vi "Cost.vi"(1 "Y":T1, 2 "Predictions":T1) -> (0 "Cost":dbl)   [LabVIEW 2016]
uses:
  <vilib>/Analysis/Matrix/Datatypes/RealMatrix.ctl
  <vilib>/Analysis/7linalg.llb/Real Transpose Matrix.vi
  <vilib>/Analysis/Matrix/Numeric/Conversions/Matrix To Array - RM.vi
  <vilib>/Analysis/Matrix/Numeric/Conversions/Array To Matrix - RA2.vi
  <vilib>/Analysis/Matrix/Numeric/Multiply/Multiply - RM,RM.vi
  <vilib>/Analysis/Matrix/Numeric/Subtract/Subtract (Elementwise) - R,RM.vi
  <vilib>/Analysis/Matrix/Numeric/Add/Add - RM,RM.vi
  <vilib>/Analysis/Matrix/Numeric/Multiply/Multiply - RM,R.vi
  <vilib>/Analysis/Matrix/NI_Matrix.lvlib
  <vilib>/Analysis/NI_AALPro.lvlib
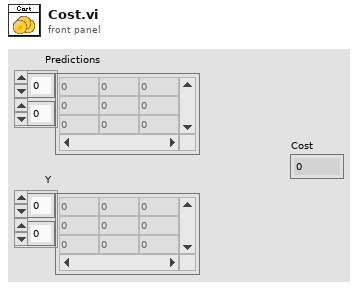
[diagram p1: front panel]
types:
  T1 = typedef "NI_Matrix.lvlib/RealMatrix.ctl" = dbl[][]
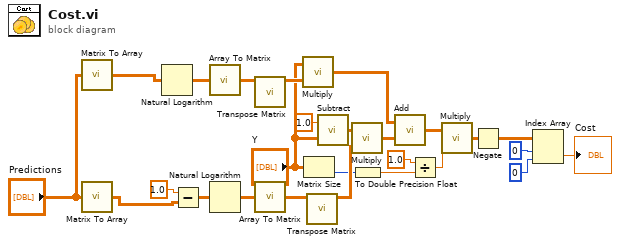
[diagram p0: block diagram]
diagram:
  n1 = call-poly <vilib>:"Matrix To Array.vi"("Real Matrix"="Predictions") -> ("Real 2D Array"=w1:dbl[][])
  n2 = call-poly <vilib>:"Matrix To Array.vi"("Real Matrix"="Predictions") -> ("Real 2D Array"=w3:dbl[][])
  n3 = Natural Logarithm(1:w1) -> (0:w26:dbl[][])
  n4 = Subtract(x=1.0, y=w3) -> (x-y=w2:dbl[][])
  n5 = call-poly <vilib>:"Array To Matrix.vi"("Real 2D Array"=w26) -> ("Real Matrix"=w25:T1)
  n6 = Natural Logarithm(1:w2) -> (0:w21:dbl[][])
  n7 = call-poly <vilib>:"Transpose Matrix.vi"("Input Matrix"=w25) -> ("Matrix Transpose"=w24:T1)  [unwired: 9 in, 1 out]
  n8 = call-poly <vilib>:"Array To Matrix.vi"("Real 2D Array"=w21) -> ("Real Matrix"=w20:T1)
  n9 = call-poly <vilib>:"Multiply.vi"("Real Matrix B"=w24, "Real Matrix A"="Y") -> ("A * B"=w22:T1)
  n10 = Matrix Size(0:"Y") -> (2:w14:i32)  [unwired: 1 out]
  n11 = call-poly <vilib>:"Transpose Matrix.vi"("Input Matrix"=w20) -> ("Matrix Transpose"=w18:T1)  [unwired: 9 in, 1 out]
  n12 = call-poly <vilib>:"Subtract.vi"("Real Matrix A"="Y", "Real Scalar c"=1.0 ("x")) -> ("c - A"=w17:T1)
  n13 = call-poly <vilib>:"Multiply.vi"("Real Matrix B"=w18, "Real Matrix A"=w17) -> ("A * B"=w16:T1)
  n14 = To Double Precision Float(number=w14) -> (double precision float=w13:dbl)
  n15 = call-poly <vilib>:"Add.vi"("Real Matrix B"=w16, "Real Matrix A"=w22) -> ("A + B"=w10:T1)
  n16 = Divide(x=1.0, y=w13) -> (x/y=w9:dbl)
  n17 = call-poly <vilib>:"Multiply.vi"("Real Scalar c"=w9, "Real Matrix A"=w10) -> ("A * c"=w8:T1)
  n18 = Negate(x=w8) -> (-x=w7:T1)
  n19 = Index Array(array=w7, index (row)=0, index (col)=0) -> (element=→"Cost":dbl)
